vi "3d queue.vi"() -> ()   [LabVIEW 2023]
uses:
  control/Data Form.ctl
  control/file structure.ctl
  <vilib>/Analysis/1siggen.llb/Ramp Pattern by Samples.vi
  queue/Front Panel Message Queue.lvlib
  <vilib>/Analysis/NI_AALBase.lvlib
panel:
  out "XY Graph":cluster{"Ramp Pattern":dbl[], i32[]}(graph)
  out "Data Form":T1
  out "error out":errorcluster
  in  "error in":errorcluster
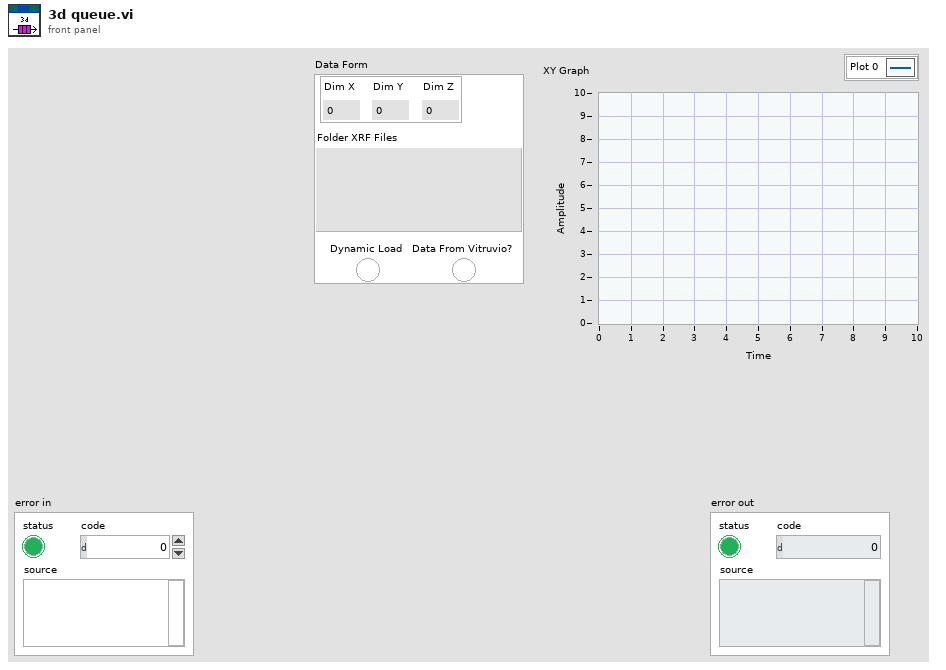
[diagram p1: front panel]
types:
  T1 = typedef "Data Form.ctl" = cluster{"Dimensions":cluster{"Dim X":i32, "Dim Y":i32, "Dim Z":i32}, "Folder XRF Files":path, "Dynamic Load":bool, "Data From Vitruvio?":bool}
  T2 = typedef "Front Panel Message Queue.lvlib/2d3d Message Queues.ctl" = cluster{"Main":refnum<queue>, "2d":refnum<queue>, "3d":refnum<queue>}
  T3 = typedef "file structure.ctl" = cluster{"Colonna":i32, "Offset Righe":i32, "Coda Righe":i32, "Transpose":bool}
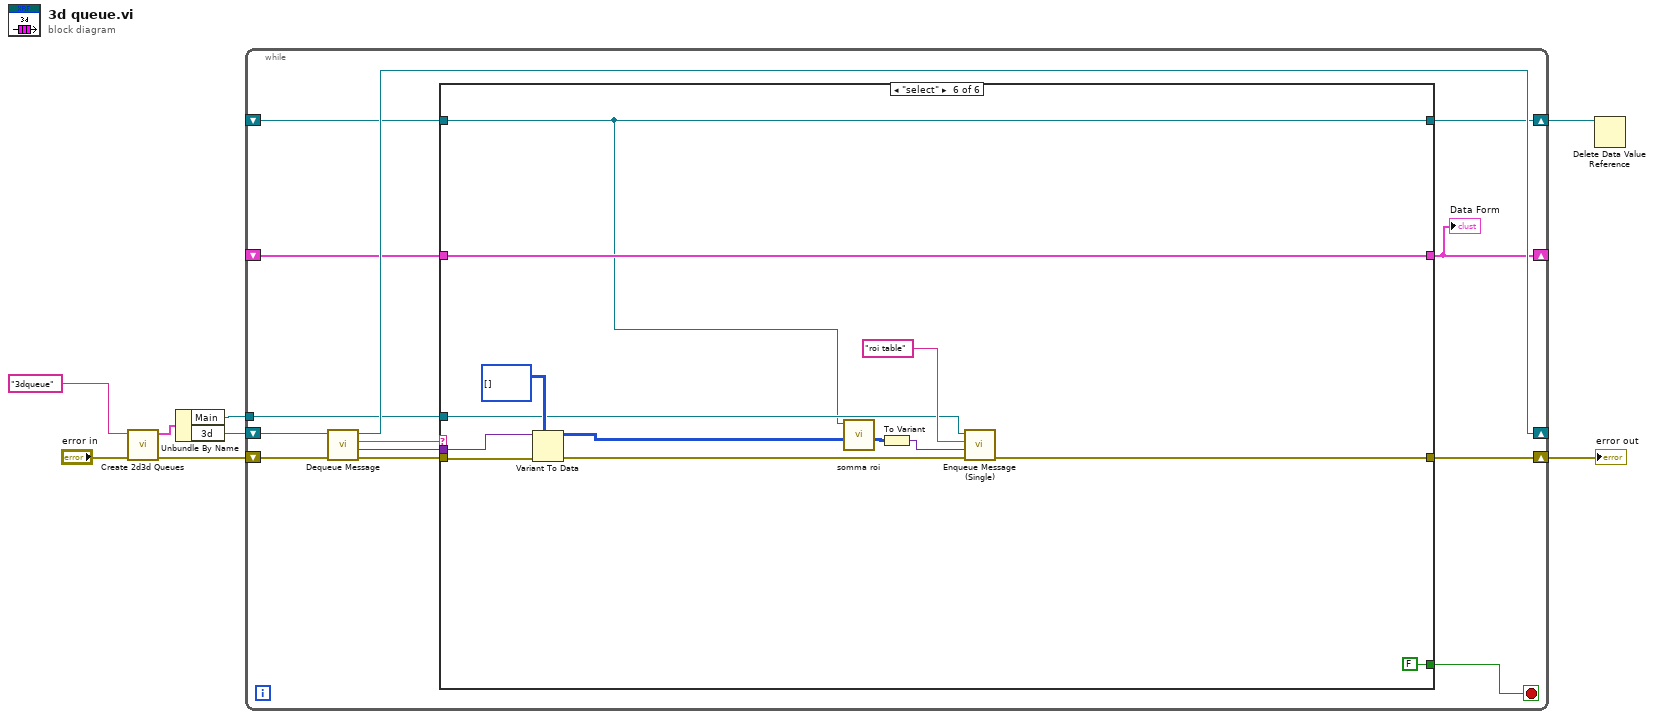
[diagram p0: block diagram]
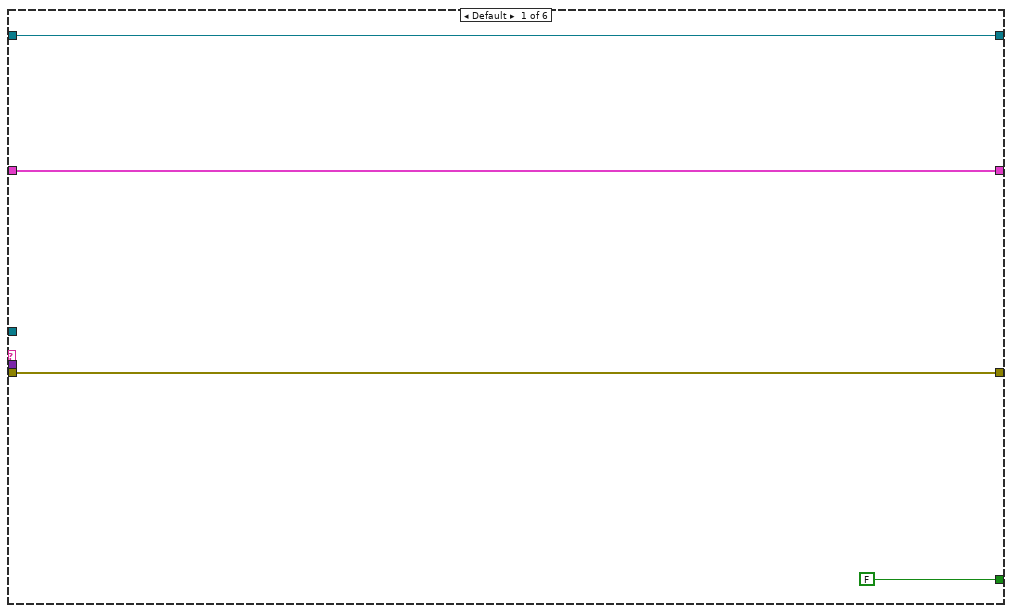
[diagram p2: hidden frame]
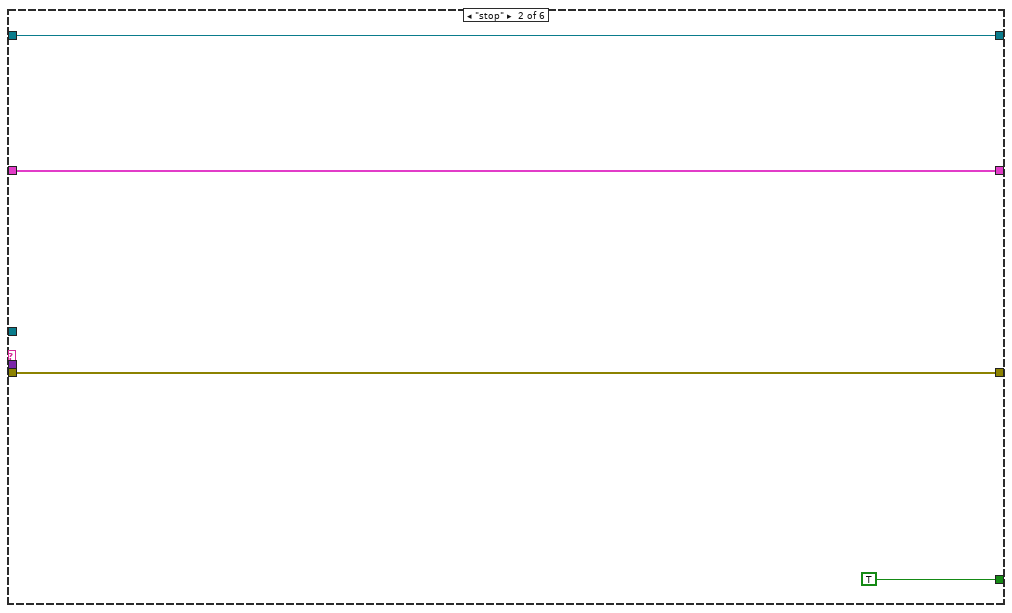
[diagram p3: hidden frame]
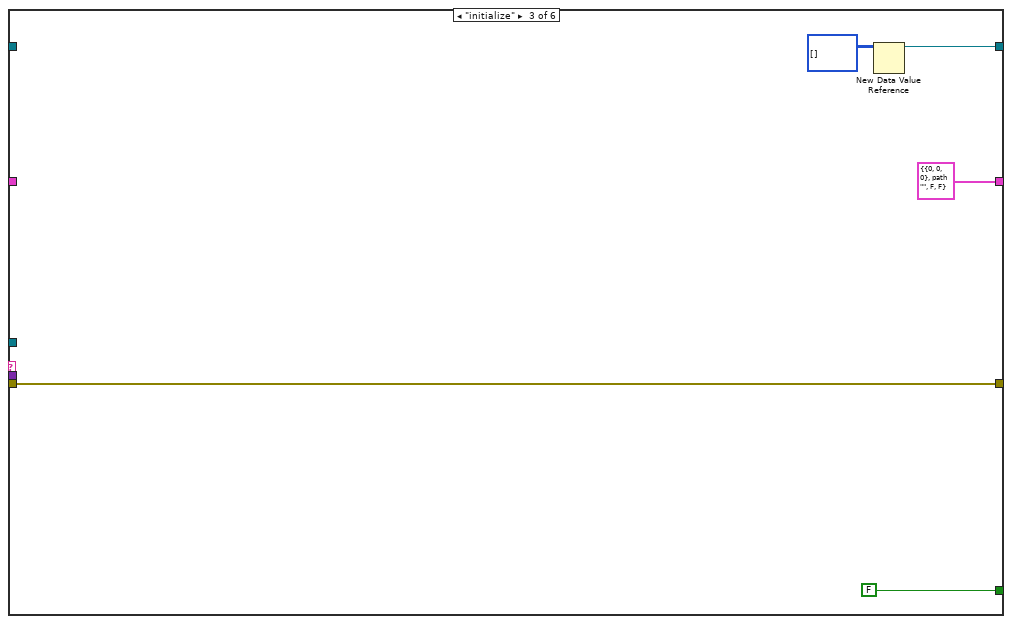
[diagram p4: hidden frame]
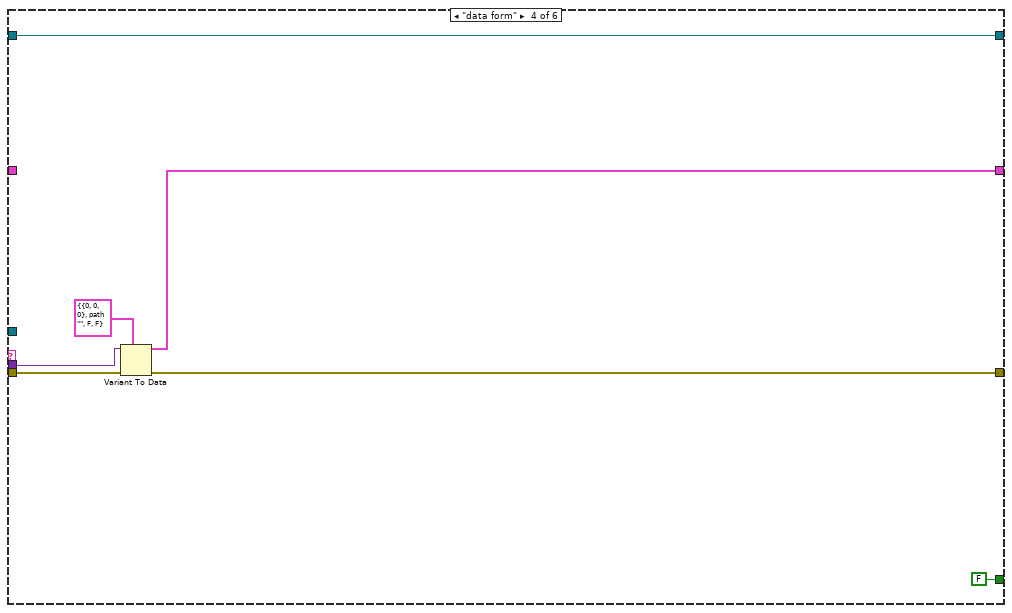
[diagram p5: hidden frame]
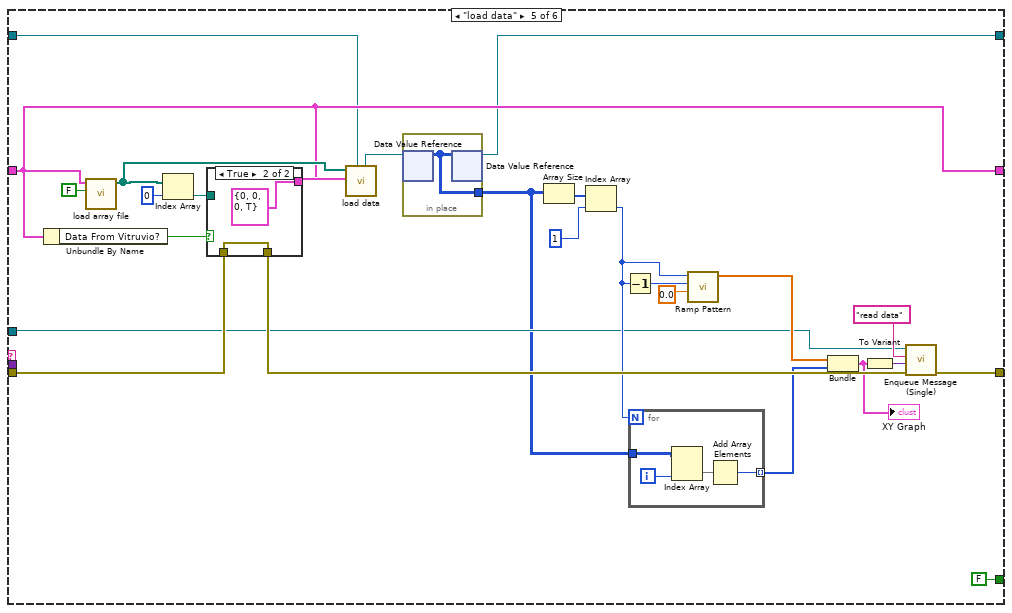
[diagram p6: hidden frame]
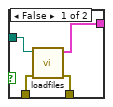
[diagram p7: hidden frame]
diagram:
  n1 = call "Create 2d3d Queues.vi"("error in (no error)"="error in", "name"="3dqueue") -> ("error out"=w4:errorcluster, "Message Queues"=w5:T2)  [unwired: 8 in]
  n2 = Unbundle By Name(w5) -> ("Main"=w2:refnum<queue>, "3d"=w8:refnum<queue>)
  n3 = while {
    shift-right: [w18] -> _
    shift-left: w8 -> [w20]
    shift-right: [w15] -> w7
    shift-left: w4 -> [w21]
    shift-right: [w13] -> _
    shift-left: _ -> [w14]
    shift-right: [w11] -> w1
    shift-left: _ -> [w10]
    tunnel: w2 -> [w9]
    stop <- w16 stop-if-true
    n4 = call "Dequeue Message.vi"("error in (no error)"=w21, "Message Queue"=w20) -> ("error out"=w19:errorcluster, "Message Data"=w12:variant, "Message"=w17:string, "dup Message Queue"=w18:refnum<queue>)  [unwired: 5 in, 1 out]
    n5 = case shown="\"select\"" w17 {
      tunnel: w19 -> [w24 w28 w33 w39 w48 w86]
      tunnel: [FALSE TRUE FALSE FALSE FALSE FALSE] -> w16
      tunnel: [w24 w28 w33 w36 w49 w83] -> w15
      tunnel: [w23 w27 T1 {"Dimensions"={"Dim X"=0, "Dim Y"=0, "Dim Z"=0}, "Folder XRF Files"=path "", "Dynamic Load"=FALSE, "Data From Vitruvio?"=FALSE} ("Data Form") w37 w46 w84] -> w13
      tunnel: w14 -> [w23 w27 _ _ w46 w84]
      tunnel: w12 -> [_ _ _ w38 _ w85]
      tunnel: [w22 w26 w30 w35 w43 w79] -> w11
      tunnel: w10 -> [w22 w26 _ w35 w44 w79]
      tunnel: w9 -> [_ _ _ _ w47 w87]
      frame Default {
      }
      frame "stop" {
      }
      frame "initialize" {
        n6 = New Data Value Reference(data value=i32[][] [] ("Data Loaded")) -> (data value reference=w30:refnum<data-value>)  [unwired: 1 in, 1 out]
      }
      frame "data form" {
        n7 = Variant To Data(error in=w39, type=T1 {"Dimensions"={"Dim X"=0, "Dim Y"=0, "Dim Z"=0}, "Folder XRF Files"=path "", "Dynamic Load"=FALSE, "Data From Vitruvio?"=FALSE} ("Data Form"), Variant=w38) -> (data=w37:T1, error out=w36:errorcluster)
      }
      frame "load data" {
        n8 = Unbundle By Name(w46) -> ("Data From Vitruvio?"=w56:bool)
        n9 = call "load array file.vi"("2d?"=FALSE, "Data Form"=w46) -> ("File Array Out"=w63:path[])  [unwired: 9 in]
        n10 = Index Array(array=w63, index=0) -> (element=w64:path)
        n11 = case shown="True" w56 {
          tunnel: w64 -> [w70 _]
          tunnel: w48 -> [w72 w74]
          tunnel: [w69 T3 {"Colonna"=0, "Offset Righe"=0, "Coda Righe"=0, "Transpose"=TRUE} ("File Structure")] -> w62
          tunnel: [w71 w74] -> w59
          frame False {
            n12 = call "loadfiles.vi"("Error In"=w72, "First Spectrum"=w70) -> ("Error Out"=w71:errorcluster, "File Structure"=w69:T3)  [unwired: 8 in]
          }
          frame True {
          }
        }
        n13 = call "load data.vi"("Data loaded reference In"=w44, "File Structure"=w62, "Data Form"=w46, "File Array In"=w63) -> ("Data loaded reference Out"=w45:refnum<data-value>)  [unwired: 7 in]
        n14 = in-place {
          in-place-border: [w68] -> w42
          n15 = in-place-dvr #1(w45) -> (w68:i32[][])  [unwired: 1 out]
          n16 = in-place-dvr #1(w68) -> (w43:refnum<data-value>)  [unwired: 1 out]
        }
        n17 = Array Size(array=w42) -> (size(s)=w61:i32[])
        n18 = Index Array(array=w61, index=1) -> (element=w53:i32)
        n19 = Decrement(x=w53) -> (x-1=w55:i32)
        n20 = for {
          N: w53 -> [_]
          tunnel: w42 -> [w77]
          tunnel: [w75] -> w51 mode=indexing
          i -> [w76]
          n21 = Index Array(array=w77, index (col)=w76) -> (element=w78:i32[])  [unwired: 1 in]
          n22 = Add Array Elements(numeric array=w78) -> (sum=w75:i32)
        }
        n23 = call-poly <vilib>:"Ramp Pattern.vi"("start"=0.0, "end"=w55, "samples"=w53) -> ("Ramp Pattern"=w52:dbl[])  [unwired: 7 in, 1 out]
        n24 = Bundle("Ramp Pattern"=w52, w51) -> (w50:cluster{"Ramp Pattern":dbl[], i32[]})  [unwired: 1 in]
        "XY Graph" <- w50
        n25 = To Variant(anything=w50) -> (Variant=w57:variant)
        n26 = call "Enqueue Message (Single).vi"("error in (no error)"=w59, "Message Data"=w57, "Message"="read data", "Message Queue"=w47) -> ("error out"=w49:errorcluster)  [unwired: 6 in, 1 out]
      }
      frame "select" {
        n27 = Variant To Data(error in=w86, type=i32[][] [] ("ROIs Min Max"), Variant=w85) -> (data=w80:i32[][], error out=w89:errorcluster)
        n28 = call "somma roi.vi"("ROIs Min Max"=w80, "Data loaded reference In"=w79) -> ("ROIs Array Out"=w81:i32[][])  [unwired: 9 in]
        n29 = To Variant(anything=w81) -> (Variant=w90:variant)
        n30 = call "Enqueue Message (Single).vi"("error in (no error)"=w89, "Message Data"=w90, "Message"="roi table", "Message Queue"=w87) -> ("error out"=w83:errorcluster)  [unwired: 6 in, 1 out]
      }
    }
    "Data Form" <- w13
  }
  "error out" <- w7
  n31 = Delete Data Value Reference(data value reference=w1) -> ()  [unwired: 1 in, 2 out]
